vi "Queue Message Handle Simple.vi"   [LabVIEW 2020]
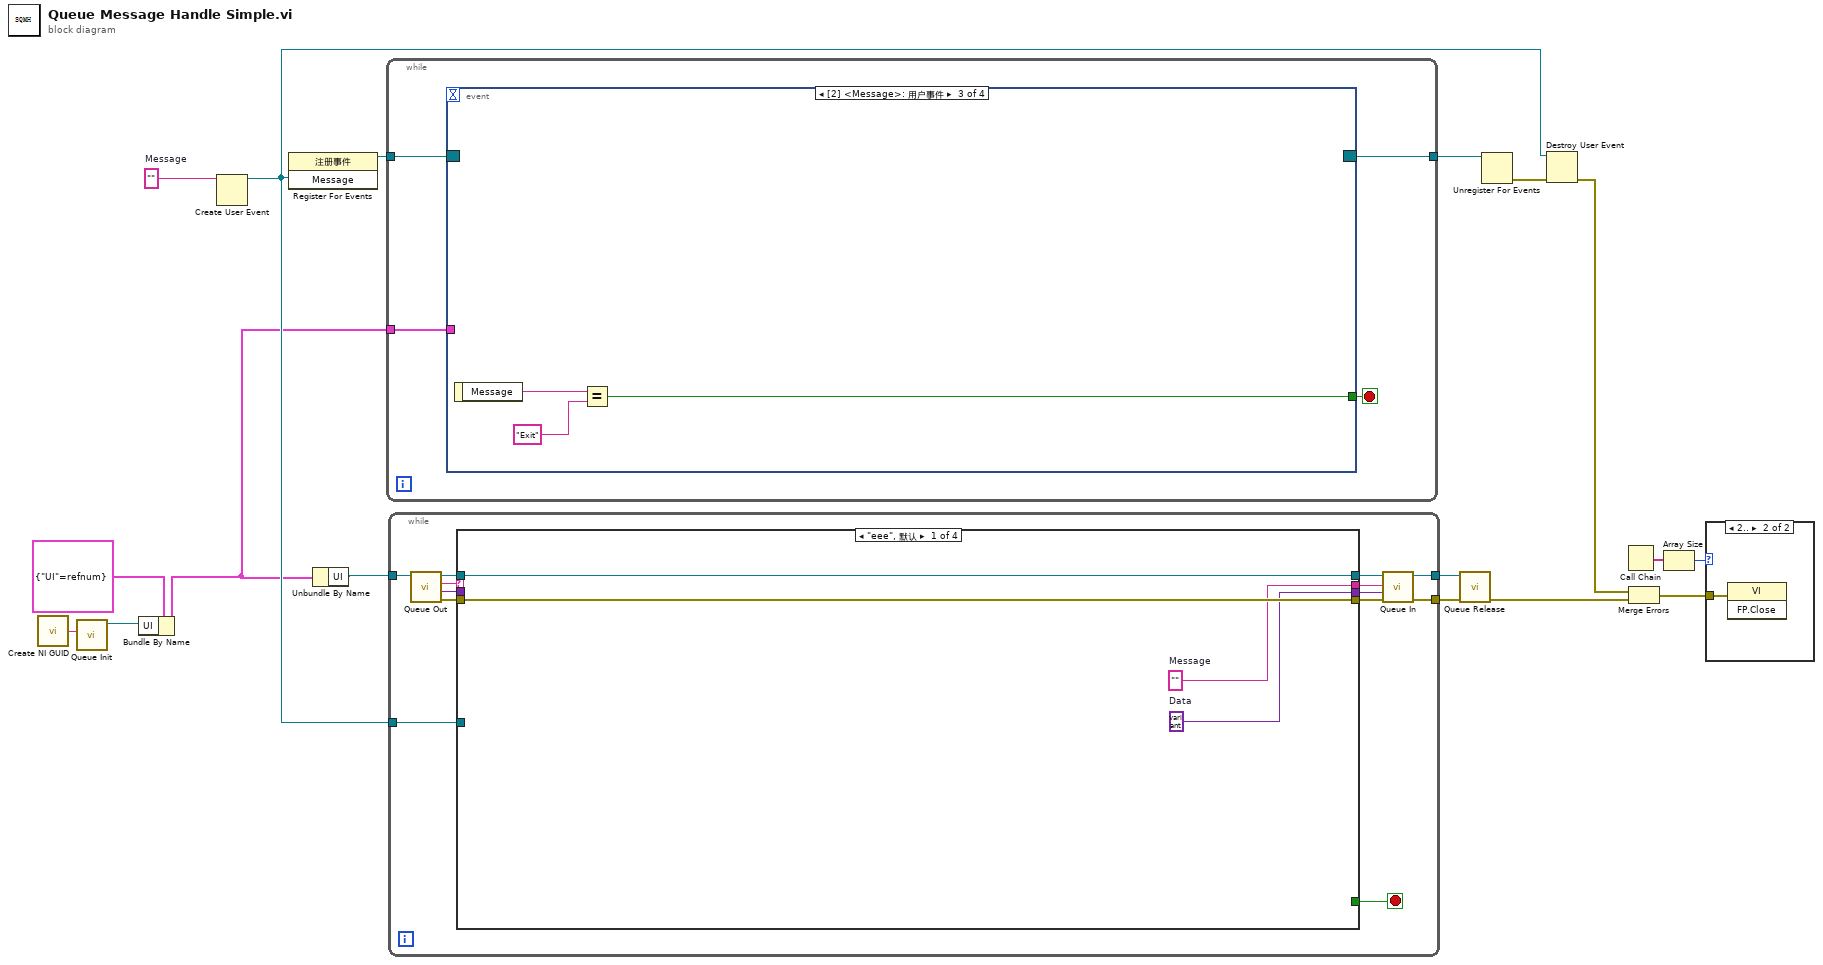
[diagram p0: block diagram]
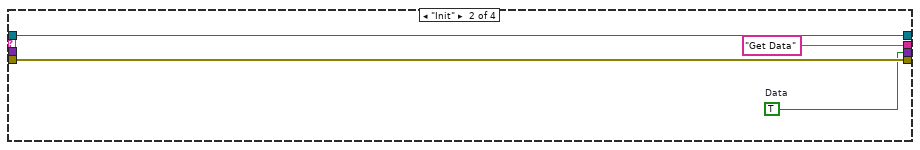
[diagram p3: hidden frame]
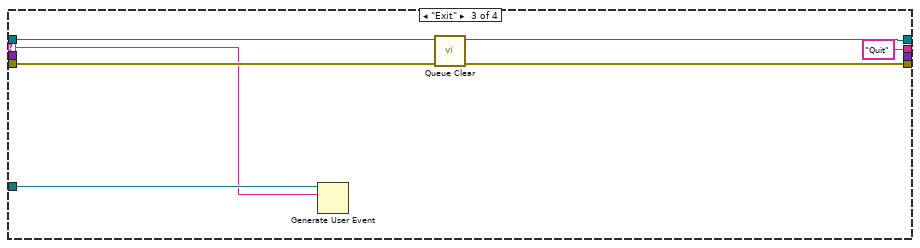
[diagram p4: hidden frame]
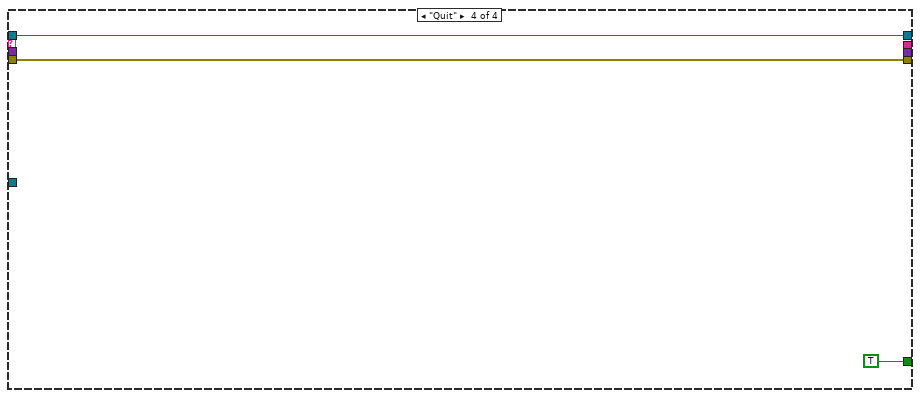
[diagram p5: hidden frame]
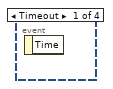
[diagram p6: hidden frame]
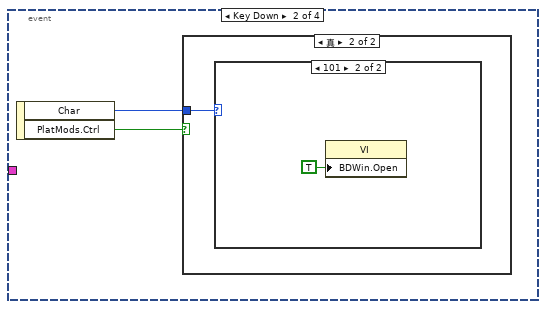
[diagram p7: hidden frame]
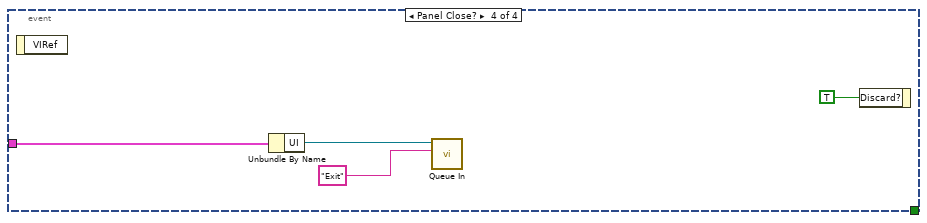
[diagram p10: hidden frame]
diagram:
  w5 = ""  # Message
  n1 = call <vilib>:"Create NI GUID.vi"() -> ("NI GUID"=w3:string)
  n2 = call "Queue Init.vi"("Queue Name"=w3) -> ("Queue Out"=w1:refnum<queue>)  [unwired: 8 in, 2 out]
  n3 = Bundle By Name(cluster=cluster{"UI":refnum<queue>} {"UI"=refnum} ("Queue Ref Out"), "UI"=w1) -> (w2:cluster{"UI":refnum<queue>})
  n4 = Create User Event(user event datatype=w5) -> (user event=w9:refnum<user-event>)  [unwired: 1 in, 1 out]
  n5 = register-events(w9) -> (reference out=w6:refnum<event-registration>)  [unwired: 2 in, 1 out]
  n6 = Unbundle By Name(w2) -> ("UI"=w12:refnum<queue>)
  n7 = while {
    tunnel: w6 -> [w21]
    tunnel: [w19] -> w7
    tunnel: w2 -> [w18]
    stop <- w20 stop-if-true
    n8 = event shown="[2] <Message>: 用户事件" {
      selector: w21 -> [_ _ _ _]
      dyn-events: [_ _ _ _] -> w19
      timeout: _ -> [_ _ _ _]
      tunnel: [_ _ w26 _] -> w20
      tunnel: w18 -> [_ _ _ w31]
      event Timeout {
        n9 = event-data() -> ()  [unwired: 1 in, 1 out]
      }
      event Key Down {
        n10 = event-data() -> ("Char"=w23:i16, "PlatMods.Ctrl"=w22:bool)  [unwired: 1 in]
        n11 = case shown="真" w22 {
          tunnel: w23 -> [_ w24]
          frame False {
          }
          frame True {
            n12 = case shown="101" w24 {
              frame 0, Default {
              }
              frame 101 {
                n13 = property class="VI"("BDWin.Open"=TRUE ("程序框图窗口:打开")) -> ()  [unwired: 2 in, 2 out]
              }
            }
          }
        }
      }
      event User Event {
        n14 = event-data() -> ("Message"=w28:string)  [unwired: 1 in]
        n15 = Equal?(x=w28, y="Exit") -> (x = y?=w26:bool)
      }
      event Panel Close? {
        n16 = event-data() -> ()  [unwired: 1 in, 1 out]
        n17 = Unbundle By Name(w31) -> ("UI"=w30:refnum<queue>)
        n18 = call "Queue In.vi"("Message"="Exit", "Queue In"=w30) -> ()  [unwired: 8 in, 2 out]
        n19 = event-data("Discard?"=TRUE ("放弃？")) -> ()  [unwired: 1 in, 1 out]
      }
    }
  }
  n20 = while {
    tunnel: w12 -> [w40]
    tunnel: [w37] -> w10
    tunnel: [w36] -> w11
    tunnel: w9 -> [w44]
    stop <- w45 stop-if-true
    n21 = call "Queue Out.vi"("Queue In"=w40) -> ("error out"=w43:errorcluster, "Data"=w41:variant, "Message"=w42:string, "Queue Out"=w39:refnum<queue>)  [unwired: 6 in, 1 out]
    n22 = case shown="\"eee\", 默认" w42 {
      selector: w42 -> [_ _ w54 _]
      tunnel: w39 -> [w49 w53 w58 w62]
      tunnel: w43 -> [w48 w52 w56 w63]
      tunnel: [w49 w53 w57 w62] -> w38
      tunnel: [w48 w52 w55 w63] -> w35
      tunnel: [w47 "Get Data" ("Message") "Quit" _] -> w34
      tunnel: [_ _ _ TRUE] -> w45
      tunnel: w44 -> [_ _ w60 _]
      tunnel: [w46 w50 _ _] -> w33
      tunnel: w41 -> [_ _ _ _]
      frame "eee", Default {
        w46 = variant  # Data
        w47 = ""  # Message
      }
      frame "Init" {
        w50 = TRUE  # Data
      }
      frame "Exit" {
        n23 = Generate User Event(user event=w60, event data cluster=w54) -> ()  [unwired: 2 in, 2 out]
        n24 = call "Queue Clear.vi"("error in (no error)"=w56, "Queue In"=w58) -> ("error out"=w55:errorcluster, "Queue Out"=w57:refnum<queue>)  [unwired: 8 in]
      }
      frame "Quit" {
      }
    }
    n25 = call "Queue In.vi"("error in (no error)"=w35, "Data"=w33, "Message"=w34, "Queue In"=w38) -> ("error out"=w36:errorcluster, "Queue Out"=w37:refnum<queue>)  [unwired: 6 in]
  }
  n26 = call "Queue Release.vi"("error in (no error)"=w11, "Queue In"=w10) -> ("error out"=w14:errorcluster)  [unwired: 9 in]
  n27 = Unregister For Events(event registration refnum=w7) -> (error out=w8:errorcluster)  [unwired: 1 in]
  n28 = Destroy User Event(user event=w9, error in=w8) -> (error out=w13:errorcluster)
  n29 = Call Chain() -> (call chain=w16:string[])
  n30 = Merge Errors(w13, w14) -> (w15:errorcluster)
  n31 = Array Size(array=w16) -> (size(s)=w17:i32)
  n32 = case shown="2.." w17 {
    tunnel: w15 -> [_ w64]
    frame 0, Default {
    }
    frame 2.. {
      n33 = invoke class="VI" method="FP.Close"(error in=w64) -> ()  [unwired: 2 in, 3 out]
    }
  }
